vi "Host__MainNew.vi"() -> ()   [LabVIEW 2018]
uses:
  HealthCheckClass/HealthCheck.lvclass
  Master/Control/TypeDef_DigitalOuts.ctl
  Libraries/TypeDef_CurrentState.ctl
  Master/DAQ/Master_DataControl.ctl
  Master/DAQ/TypeDef_cRIOData.ctl
  Master/IMU/TypeDef_IMUData.ctl
  Master/CAN/TypeDef_BMSData.ctl
  Master/CAN/TypeDef_BMS_Status.ctl
  Master/CAN/MotorController/fixedMotorData.ctl
  Master/CAN/MotorController/MotorStatus.ctl
panel:
  out "Velocity Graph":dbl(graph)
  out "Acceleration Graph":dbl(graph)
  in  "ManualBrake":bool
  in  "ForceIdle":bool
  in  "Pod Power":bool
  out "CurrentState Ind.":u16(ring)
  in  "stop":bool
  in  "Edit Table":bool
  out "HealthCheckTable":string[][](table)
  in  "Tab Control":T1
  in  "Ignition":bool
  in  "Service Toggle":bool
  in  "ServiceHOLD":bool
  in  "DrvieEnable":bool
  in  "DriveEnable(SC)":bool
  in  "High Side (SC)":bool
  in  "Pre-Charge (SC)":bool
  in  "Low Side (SC)":bool
  in  "Ignition (SC)":bool
  in  "Pump (SC)":bool
  in  "Clamp (SC)":bool
  in  "Brakes (SC)":bool
  in  "HighSidePermission (SC)":bool caption="High\nSide"
  in  "Launch":bool
  in  "Ready":bool
  in  "Pre-charge":bool
  in  "Motor Controller":bool
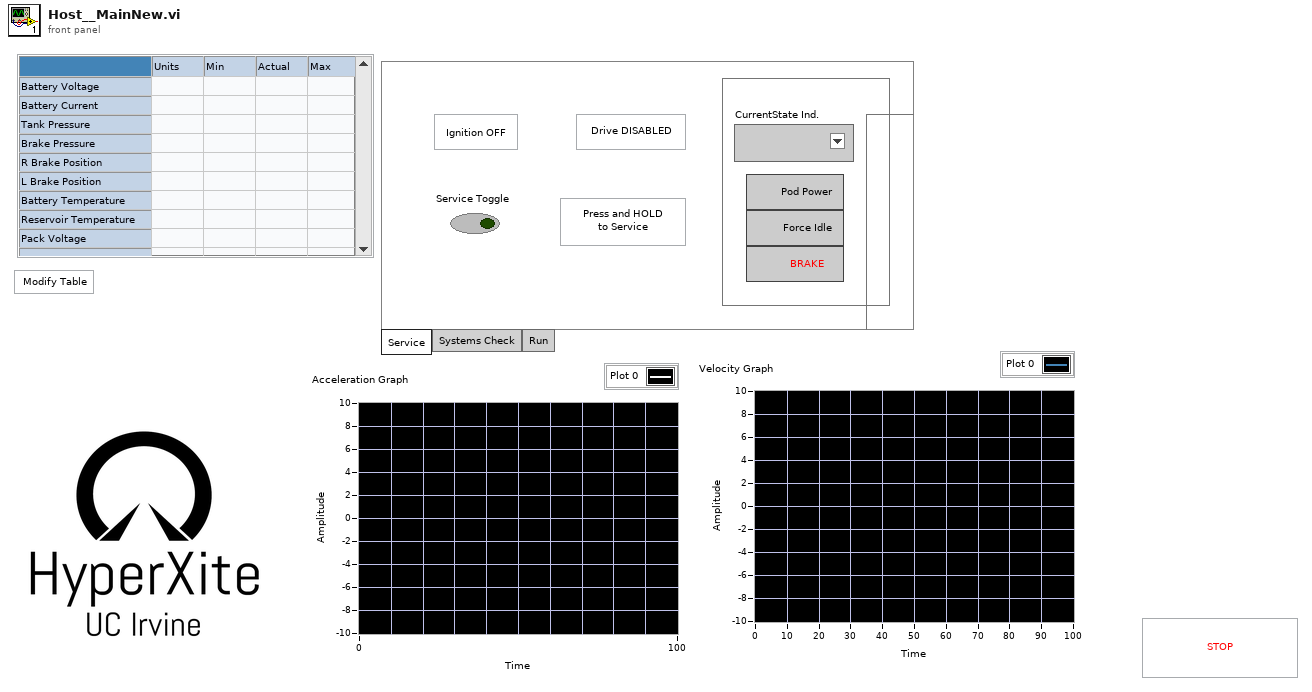
[diagram p1: front panel]
types:
  T1 = typedef "Control 2" = enum32{"Service", "Systems Check", "Run"}
  T2 = enum8{"Enabled", "Disabled", "Disabled and Grayed Out"}
  T3 = typedef "Master_DataControl.ctl" = cluster{"cRIO Data":T4, "IMU Data":T5, "BMS Data":T6, "Motor Data":T8}
  T4 = typedef "TypeDef_cRIOData.ctl" = cluster{"Time (ms)":dbl, "24V Battery (V)":dbl, "LowV Current (A)":dbl, "Fiducial Sensor (V)":dbl, "PV Pressure (psig)":dbl, "Flow Sensor (V)":dbl, "Temp Fairing (F)":dbl, "Temp Reservoir (F)":dbl, "HallEffect Right (in)":dbl, "HallEffect Left (in)":dbl, "PT Tank (psig)":dbl, "PT Clamp Right (psig)":dbl, "PT Clamp Left (psig)":dbl, "PT Brake (psig)":dbl, "PT Cooling (psig)":dbl, "Displacement (ft)":dbl, "Velocity (ft/s)":dbl}
  T5 = typedef "TypeDef_IMUData.ctl" = cluster{"x acceleration (g)":dbl, "Pressure (psia)":dbl, "Temperature (F)":dbl}
  T6 = typedef "TypeDef_BMSData.ctl" = cluster{"Max Cell Voltage (V)":dbl, "Max Cell ID":dbl, "Min Cell Voltage (V)":dbl, "Min Cell ID":dbl, "State of Charge (%)":dbl, "Average Voltage (V)":dbl, "Voltage Delta (V)":dbl, "Pack Current (A)":dbl, "Pack Voltage (V)":dbl, "Max Resistance (Ohm)":dbl, "Min Resistance (Ohm)":dbl, "Average Resistance (Ohm)":dbl, "Delta Resistance (Ohm)":dbl, "Highest Temperature(F)":dbl, "BmsStatus":T7}
  T7 = typedef "TypeDef_BMS_Status.ctl" = cluster{"isFault":bool, "isolationMonitoring":bool}
  T8 = typedef "fixedMotorData.ctl" = cluster{"Velo (RPM)":dbl, "MotorTemp(F)":dbl, "CtrlTemp(F)":dbl, "DcLinkVolt(V)":dbl, "ErrorCode":dbl, "motorStatus":T9, "isAlive":bool, "motorControllerState":u16}
  T9 = typedef "MotorStatus.ctl" = cluster{"isReady":bool, "isOn":bool, "isOperEn":bool, "isFault":bool, "isVoltEn":bool, "targetReached":bool, "isWarning":bool}
  T10 = typedef "TypeDef_CurrentState.ctl" = enum16{"Fault", "Idle", "Ready", "Pushing", "Coast", "Braking"}
  T11 = typedef "TypeDef_DigitalOuts.ctl" = cluster{"Pod Power":bool, "Dump Valve":bool, "Brakes":bool, "Clamp":bool, "Pump":bool, "Ignition":bool, "DO6":bool, "DO7":bool, "HighSide":bool, "Precharge":bool, "LowSide":bool, "DO3":bool, "DO4":bool, "DO5":bool, "DO62":bool, "DO72":bool}
  T12 = typedef "HealthCheck.lvclass/HCState_TypeDef.ctl" = enum16{"Initialization", "Running", "Modify Table"}
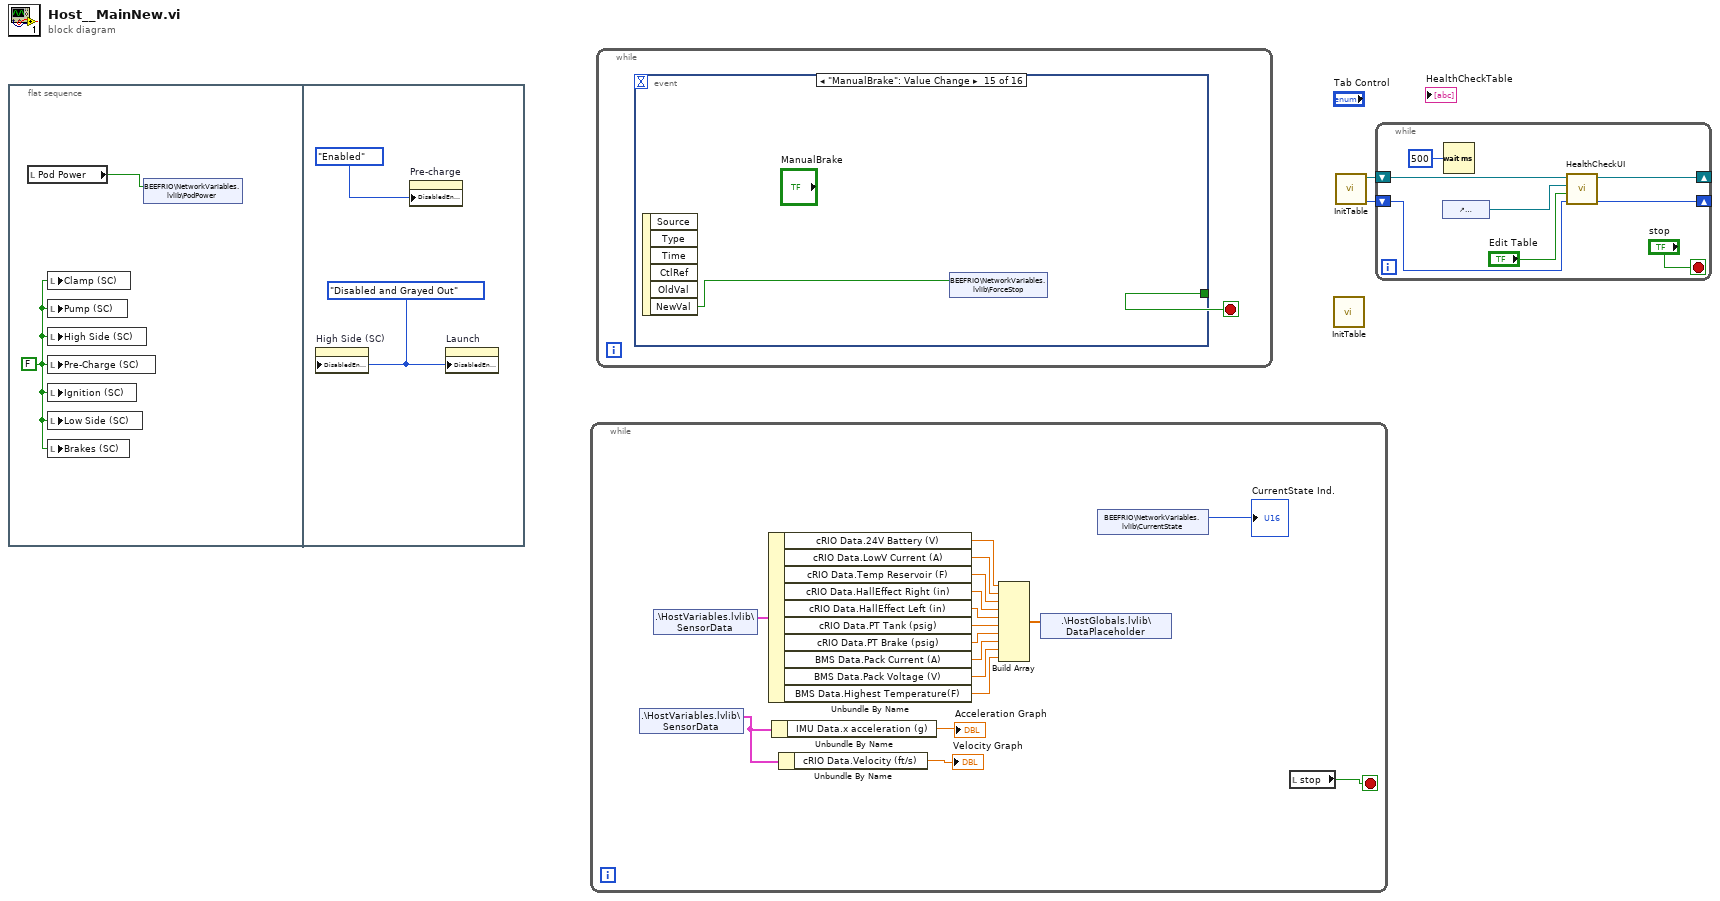
[diagram p0: block diagram]
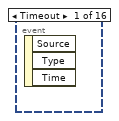
[diagram p2: hidden frame]
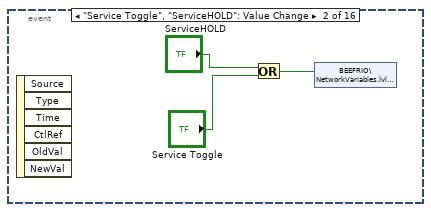
[diagram p3: hidden frame]
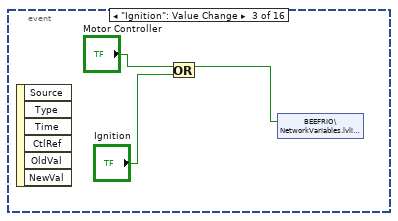
[diagram p4: hidden frame]
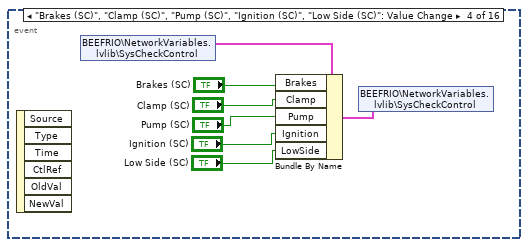
[diagram p5: hidden frame]
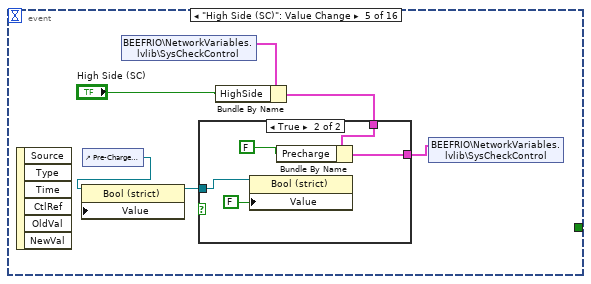
[diagram p6: hidden frame]
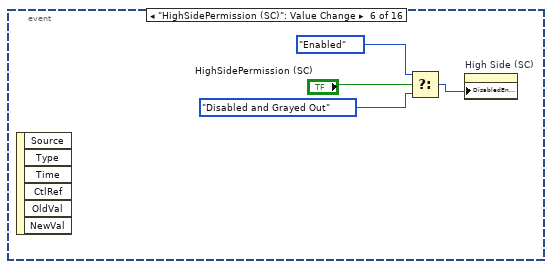
[diagram p8: hidden frame]
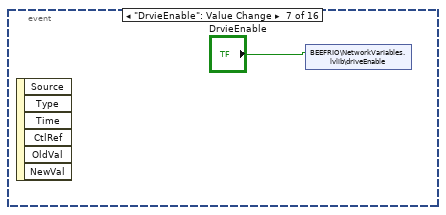
[diagram p9: hidden frame]
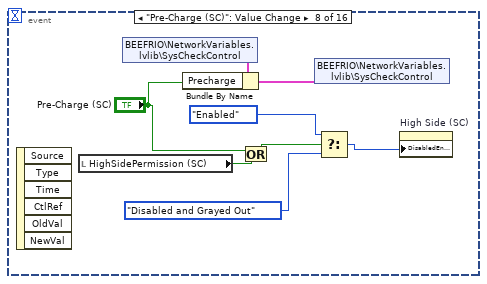
[diagram p10: hidden frame]
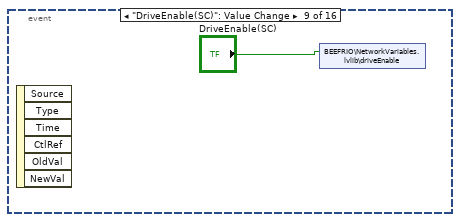
[diagram p11: hidden frame]
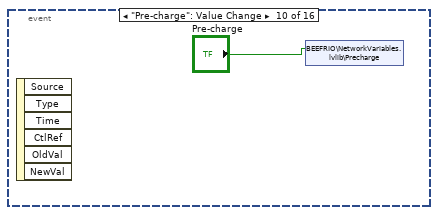
[diagram p12: hidden frame]
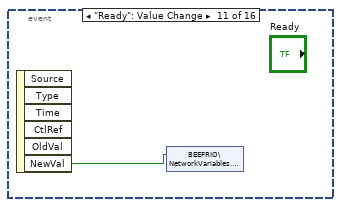
[diagram p13: hidden frame]
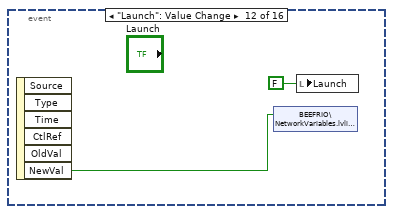
[diagram p14: hidden frame]
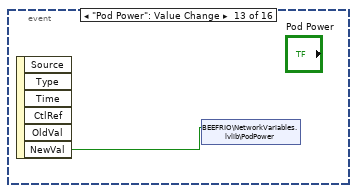
[diagram p15: hidden frame]
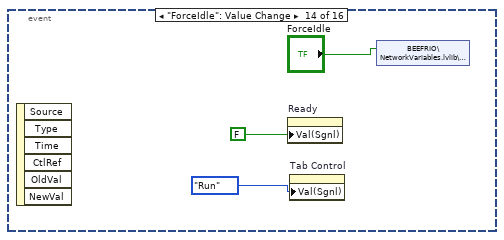
[diagram p16: hidden frame]
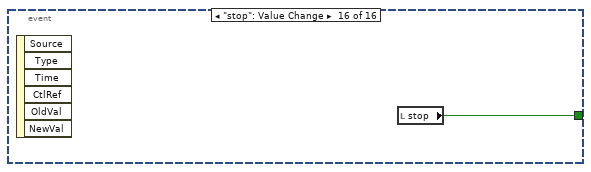
[diagram p17: hidden frame]
diagram:
  n1 = flat-sequence {
    frame #0 {
      w3 = FALSE
      n2 = local read "Pod Power"() -> (w4:bool)
      n3 = local write "Clamp (SC)"(w3) -> ()
      n4 = local write "Pump (SC)"(w3) -> ()
      n5 = local write "High Side (SC)"(w3) -> ()
      n6 = local write "Pre-Charge (SC)"(w3) -> ()
      n7 = local write "Ignition (SC)"(w3) -> ()
      n8 = local write "Low Side (SC)"(w3) -> ()
      n9 = local write "Brakes (SC)"(w3) -> ()
      n10 = shared-variable "BEEFRIO\\NetworkVariables.lvlib\\PodPower"(w4) -> ()  [unwired: 1 in, 1 out]
    }
    frame #1 {
      w5 = T2."Disabled and Grayed Out" ("Disabled")
      n11 = property on="High Side (SC)" class="Bool (strict)"("DisabledEnum"=w5) -> ()  [unwired: 2 in, 2 out]
      n12 = property on="Pre-charge" class="Bool"("DisabledEnum"=T2."Enabled" ("Disabled")) -> ()  [unwired: 2 in, 2 out]
      n13 = property on="Launch" class="Bool"("DisabledEnum"=w5) -> ()  [unwired: 2 in, 2 out]
    }
  }
  n14 = while {
    stop <- w11 stop-if-true
    n15 = shared-variable ".\\HostVariables.lvlib\\SensorData"() -> (w8:T3)  [unwired: 1 in, 1 out]
    n16 = shared-variable ".\\HostVariables.lvlib\\SensorData"() -> (w23:T3)  [unwired: 1 in, 1 out]
    n17 = Unbundle By Name(w23) -> ("cRIO Data.24V Battery (V)"=w22:dbl, "cRIO Data.LowV Current (A)"=w21:dbl, "cRIO Data.Temp Reservoir (F)"=w20:dbl, "cRIO Data.HallEffect Right (in)"=w19:dbl, "cRIO Data.HallEffect Left (in)"=w18:dbl, "cRIO Data.PT Tank (psig)"=w17:dbl, "cRIO Data.PT Brake (psig)"=w16:dbl, "BMS Data.Pack Current (A)"=w15:dbl, "BMS Data.Pack Voltage (V)"=w14:dbl, "BMS Data.Highest Temperature(F)"=w13:dbl)
    n18 = Unbundle By Name(w8) -> ("IMU Data.x acceleration (g)"=→"Acceleration Graph":dbl)
    n19 = Unbundle By Name(w8) -> ("cRIO Data.Velocity (ft/s)"=→"Velocity Graph":dbl)
    n20 = Build Array(w22, w21, w20, w19, w18, w17, w16, w15, w14, w13) -> (w12:dbl[])
    n21 = shared-variable ".\\HostGlobals.lvlib\\DataPlaceholder"(w12) -> ()  [unwired: 1 in, 1 out]
    n22 = shared-variable "BEEFRIO\\NetworkVariables.lvlib\\CurrentState"() -> (→"CurrentState Ind.":T10)  [unwired: 1 in, 1 out]
    n23 = local read "stop"() -> (w11:bool)
  }
  n24 = while {
    stop <- w24 stop-if-true
    n25 = event shown="[14] \"ManualBrake\": Value Change" {
      selector: _ -> [_ _ _ _ _ _ _ _ _ _ _ _ _ _ _ _]
      dyn-events: _ -> [_ _ _ _ _ _ _ _ _ _ _ _ _ _ _ _]
      timeout: _ -> [_ _ _ _ _ _ _ _ _ _ _ _ _ _ _ _]
      tunnel: [_ _ _ _ _ _ _ _ _ _ _ _ _ _ _ w73] -> w24
      event Timeout {
        n26 = event-data() -> ()  [unwired: 1 in, 3 out]
      }
      event "Service Toggle", "ServiceHOLD": Value Change {
        n27 = event-data() -> ()  [unwired: 1 in, 6 out]
        n28 = Or(x="ServiceHOLD", y="Service Toggle") -> (x .or. y?=w27:bool)
        n29 = shared-variable "BEEFRIO\\NetworkVariables.lvlib\\Service"(w27) -> ()  [unwired: 1 in, 1 out]
      }
      event "Ignition": Value Change {
        n30 = event-data() -> ()  [unwired: 1 in, 6 out]
        n31 = Or(x="Motor Controller", y="Ignition") -> (x .or. y?=w30:bool)
        n32 = shared-variable "BEEFRIO\\NetworkVariables.lvlib\\Ignition"(w30) -> ()  [unwired: 1 in, 1 out]
      }
      event "Brakes (SC)", "Clamp (SC)", "Pump (SC)", "Ignition (SC)", "Low Side (SC)": Value Change {
        n33 = event-data() -> ()  [unwired: 1 in, 6 out]
        n34 = shared-variable "BEEFRIO\\NetworkVariables.lvlib\\SysCheckControl"() -> (w31:T11)  [unwired: 1 in, 1 out]
        n35 = Bundle By Name(cluster=w31, "Brakes"="Brakes (SC)", "Clamp"="Clamp (SC)", "Pump"="Pump (SC)", "Ignition"="Ignition (SC)", "LowSide"="Low Side (SC)") -> (w32:T11)
        n36 = shared-variable "BEEFRIO\\NetworkVariables.lvlib\\SysCheckControl"(w32) -> ()  [unwired: 1 in, 1 out]
      }
      event "High Side (SC)": Value Change {
        n37 = event-data() -> ()  [unwired: 1 in, 6 out]
        n38 = control-ref of="Pre-Charge (SC)"() -> (w42:refnum<vi>)
        n39 = property class="Bool (strict)" props=["Value"](reference=w42) -> (reference out=w41:refnum<vi>)  [unwired: 2 in, 1 out]
        n40 = shared-variable "BEEFRIO\\NetworkVariables.lvlib\\SysCheckControl"() -> (w43:T11)  [unwired: 1 in, 1 out]
        n41 = Bundle By Name(cluster=w43, "HighSide"="High Side (SC)") -> (w40:T11)
        n42 = case shown="True" {
          selector: _ -> [_ _]
          tunnel: w41 -> [_ w48]
          tunnel: w40 -> [w44 w46]
          tunnel: [w44 w45] -> w39
          frame False {
          }
          frame True {
            n43 = property class="Bool (strict)"(reference=w48, "Value"=FALSE) -> ()  [unwired: 1 in, 2 out]
            n44 = Bundle By Name(cluster=w46, "Precharge"=FALSE ("Actuators.PrechargeContactor")) -> (w45:T11)
          }
        }
        n45 = shared-variable "BEEFRIO\\NetworkVariables.lvlib\\SysCheckControl"(w39) -> ()  [unwired: 1 in, 1 out]
      }
      event "HighSidePermission (SC)": Value Change {
        n46 = event-data() -> ()  [unwired: 1 in, 6 out]
        n47 = Select(t=T2."Enabled" ("Disabled"), s="HighSidePermission (SC)", f=T2."Disabled and Grayed Out" ("Disabled")) -> (s? t:f=w50:T2)
        n48 = property on="High Side (SC)" class="Bool (strict)"("DisabledEnum"=w50) -> ()  [unwired: 2 in, 2 out]
      }
      event "DrvieEnable": Value Change {
        n49 = event-data() -> ()  [unwired: 1 in, 6 out]
        n50 = shared-variable "BEEFRIO\\NetworkVariables.lvlib\\driveEnable"("DrvieEnable") -> ()  [unwired: 1 in, 1 out]
      }
      event "Pre-Charge (SC)": Value Change {
        n51 = event-data() -> ()  [unwired: 1 in, 6 out]
        n52 = local read "HighSidePermission (SC)"() -> (w59:bool)
        n53 = shared-variable "BEEFRIO\\NetworkVariables.lvlib\\SysCheckControl"() -> (w62:T11)  [unwired: 1 in, 1 out]
        n54 = Bundle By Name(cluster=w62, "Precharge"="Pre-Charge (SC)") -> (w61:T11)
        n55 = Or(x="Pre-Charge (SC)", y=w59) -> (x .or. y?=w60:bool)
        n56 = shared-variable "BEEFRIO\\NetworkVariables.lvlib\\SysCheckControl"(w61) -> ()  [unwired: 1 in, 1 out]
        n57 = Select(t=T2."Enabled" ("Disabled"), s=w60, f=T2."Disabled and Grayed Out" ("Disabled")) -> (s? t:f=w56:T2)
        n58 = property on="High Side (SC)" class="Bool (strict)"("DisabledEnum"=w56) -> ()  [unwired: 2 in, 2 out]
      }
      event "DriveEnable(SC)": Value Change {
        n59 = event-data() -> ()  [unwired: 1 in, 6 out]
        n60 = shared-variable "BEEFRIO\\NetworkVariables.lvlib\\driveEnable"("DriveEnable(SC)") -> ()  [unwired: 1 in, 1 out]
      }
      event "Pre-charge": Value Change {
        n61 = event-data() -> ()  [unwired: 1 in, 6 out]
        n62 = shared-variable "BEEFRIO\\NetworkVariables.lvlib\\Precharge"("Pre-charge") -> ()  [unwired: 1 in, 1 out]
      }
      event "Ready": Value Change {
        n63 = event-data() -> ("NewVal"=w65:bool)  [unwired: 1 in, 5 out]
        n64 = shared-variable "BEEFRIO\\NetworkVariables.lvlib\\Ready"(w65) -> ()  [unwired: 1 in, 1 out]
      }
      event "Launch": Value Change {
        n65 = event-data() -> ("NewVal"=w66:bool)  [unwired: 1 in, 5 out]
        n66 = shared-variable "BEEFRIO\\NetworkVariables.lvlib\\Launch"(w66) -> ()  [unwired: 1 in, 1 out]
        n67 = local write "Launch"(FALSE ("Ready")) -> ()
      }
      event "Pod Power": Value Change {
        n68 = event-data() -> ("NewVal"=w68:bool)  [unwired: 1 in, 5 out]
        n69 = shared-variable "BEEFRIO\\NetworkVariables.lvlib\\PodPower"(w68) -> ()  [unwired: 1 in, 1 out]
      }
      event "ForceIdle": Value Change {
        n70 = event-data() -> ()  [unwired: 1 in, 6 out]
        n71 = property on="Ready" class="Bool"("Val(Sgnl)"=FALSE) -> ()  [unwired: 2 in, 2 out]
        n72 = property on="Tab Control" class="TabCtl (strict)"("Val(Sgnl)"=Control_2."Run" ("Tab Control")) -> ()  [unwired: 2 in, 2 out]
        n73 = shared-variable "BEEFRIO\\NetworkVariables.lvlib\\ForceIdle"("ForceIdle") -> ()  [unwired: 1 in, 1 out]
      }
      event "ManualBrake": Value Change {
        n74 = event-data() -> ("NewVal"=w72:bool)  [unwired: 1 in, 5 out]
        n75 = shared-variable "BEEFRIO\\NetworkVariables.lvlib\\ForceStop"(w72) -> ()  [unwired: 1 in, 1 out]
      }
      event "stop": Value Change {
        n76 = event-data() -> ()  [unwired: 1 in, 6 out]
        n77 = local read "stop"() -> (w73:bool)
      }
    }
  }
  n78 = call "InitTable.vi"() -> ()  [unwired: 10 in, 2 out]
  n79 = call "InitTable.vi"() -> ("Enum out"=w1:T12, "HealthCheck out"=w2:refnum<class "HealthCheck.lvclass">)  [unwired: 10 in]
  n80 = while {
    shift-right: [w77] -> _
    shift-left: w2 -> [w76]
    shift-right: [w75] -> _
    shift-left: w1 -> [w74]
    stop <- "stop" stop-if-true
    n81 = control-ref of="HealthCheckTable"() -> (w78:refnum<vi>)
    n82 = Wait (ms)(milliseconds to wait=u32 500) -> ()  [unwired: 1 out]
    n83 = call "HealthCheckUI.vi"("Enum in"=w74, "Edit Table"="Edit Table", "Table in"=w78, "HealthCheck.lvclass"=w76) -> ("Enum out"=w75:T12, "HealthCheck out"=w77:refnum<class "HealthCheck.lvclass">)  [unwired: 6 in]
  }
